vi "snapperEventsFunctionalGlobal.vi"(9 "snapperEvents":T1, 11 "Action":enum16{"Write", "Read"}(ring)) -> (1 "snapperEvents":T1)   [LabVIEW 2009, in "Views.lvlib" / "Camera.lvlib"]
uses:
  Camera.lvlib
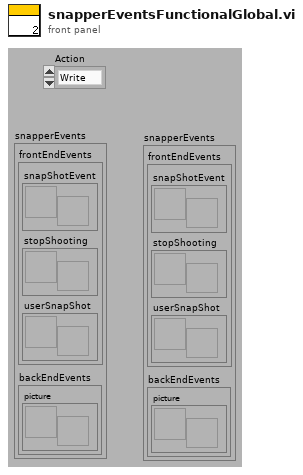
[diagram p1: front panel]
types:
  T1 = cluster{"frontEndEvents":cluster{"snapShotEvent":refnum<user-event>, "stopShooting":refnum<user-event>, "userSnapShot":refnum<user-event>}, "backEndEvents":cluster{"picture":refnum<user-event>}}
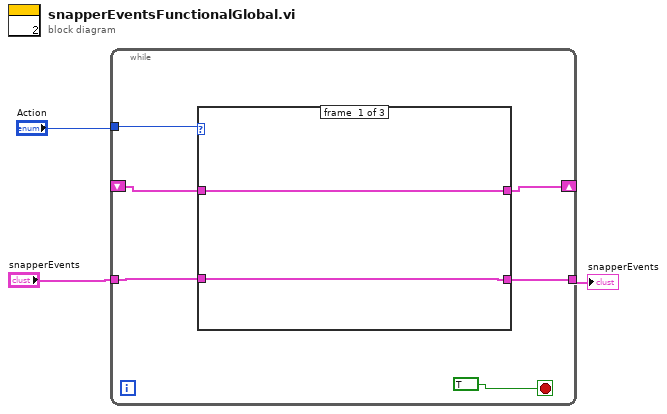
[diagram p0: block diagram]
diagram:
  n1 = while {
    tunnel: "Action" -> [w9]
    shift-right: [w5] -> _
    shift-left: _ -> [w7]
    tunnel: [w6] -> w1
    tunnel: "snapperEvents" -> [w4]
    stop <- TRUE stop-if-true
    n2 = case shown="\"Read\"" w9 {
      tunnel: [w11 w12 w13] -> w5
      tunnel: w4 -> [w10 w12 _]
      tunnel: w7 -> [w11 _ w13]
      tunnel: [w10 w12 w13] -> w6
      frame #0 {
      }
      frame #1 {
      }
      frame #2 {
      }
    }
  }
  "snapperEvents" <- w1
